vi "averI.vi"(1 "I'":dbl[][](array[numeric]), 2 "N":dbl, 3 "物体大小":i32) -> (0 "<I>":dbl[](array[numeric]))   [LabVIEW 2018]
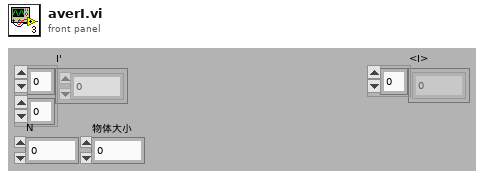
[diagram p1: front panel]
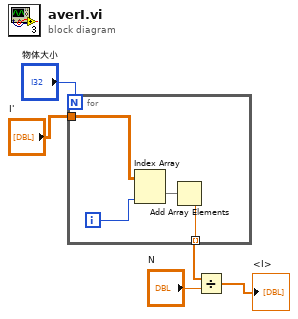
[diagram p0: block diagram]
diagram:
  n1 = for {
    N: "物体大小" -> [_]
    tunnel: [w8] -> w5 mode=indexing
    tunnel: "I'" -> [w7]
    i -> [w9]
    n2 = Index Array(array=w7, index (col)=w9) -> (element=w6:dbl[])  [unwired: 1 in]
    n3 = Add Array Elements(numeric array=w6) -> (sum=w8:dbl)
  }
  n4 = Divide(x=w5, y="N") -> (x/y=→"<I>":dbl[])
